vi "Apply Trigger Settings.vi"(8 "error in":errorcluster, 11 "4300 in":refnum<class "4300.lvclass">) -> (0 "error out":errorcluster, 3 "4300 out":refnum<class "4300.lvclass">)   [LabVIEW 2019, in "4300.lvlib" / "4300.lvclass"]
uses:
  Library/4300.lvclass
  C:/Users/Public/Documents/Development/builds/Instruments/AnalogInput.lvlibp/Library/AnalogInput.lvclass
  Library/4300.lvclass/4300.ctl
  builds/Instruments/AnalogInput.lvlibp/Accessors/Triggering/Read Trigger Source.vi
  builds/Instruments/AnalogInput.lvlibp/Accessors/Triggering/Read Trigger Settings.vi
  <vilib>/DAQmx/configure/trigger.llb/DAQmx Reference Trigger (Analog Edge).vi
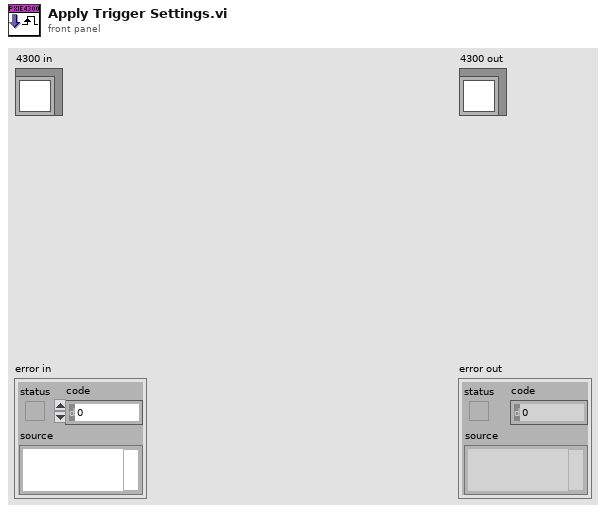
[diagram p1: front panel]
types:
  T1 = typedef "AnalogInput.lvlibp/AnalogInput.lvclass/User Trigger Settings.ctl" = cluster{"Timeout":dbl, "Level":dbl, "Slope":T2, "samples per channel":i32, "Sample Rate (10k)":dbl, "pretrigger samples":u32}
  T2 = typedef "AnalogInput.lvlibp/AnalogInput.lvclass/Trigger_Slope.ctl" = enum16{"Rising", "Falling"}
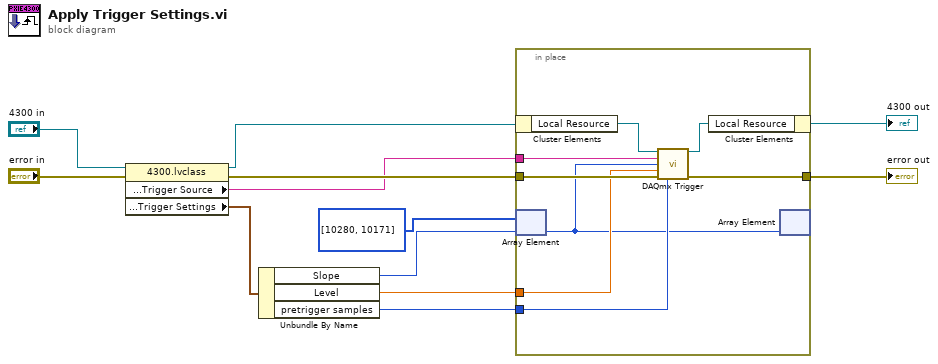
[diagram p0: block diagram]
diagram:
  w2 = i32[] [10280, 10171] items=["Rising"=10280, "Falling"=10171]
  n1 = property class="4300.lvclass"(reference="4300 in", error in="error in") -> (reference out=w4:refnum<class "4300.lvclass">, error out=w10:errorcluster, "Accessors:Triggering:Trigger Source"=w5:string, "Accessors:Triggering:Trigger Settings"=w6:T1)
  n2 = Unbundle By Name(w6) -> ("Slope"=w1:T2, "Level"=w8:dbl, "pretrigger samples"=w7:u32)
  n3 = in-place {
    in-place-border: w10 -> [w20]
    in-place-border: [w19] -> w9
    in-place-border: w8 -> [w18]
    in-place-border: w7 -> [w17]
    in-place-border: w5 -> [w16]
    n4 = in-place-cluster #1(w4) -> ("Local Resource"=w15:refnum<k21>)
    n5 = in-place-array #2(w2, w1) -> (w13:i32)
    n6 = call-poly <vilib>:"DAQmx Trigger.vi"("task/channels in"=w15, "source"=w16, "slope"=w13, "level"=w18, "error in"=w20, "pretrigger samples per channel"=w17) -> ("task out"=w14:refnum<k21>, "error out"=w19:errorcluster)  [unwired: 8 in]
    n7 = in-place-cluster #1("Local Resource"=w14) -> (→"4300 out":refnum<class "4300.lvclass">)
    n8 = in-place-array #2(w13) -> ()  [unwired: 2 out]
  }
  "error out" <- w9
